vi "DataQuery.vi"(8 "Error In":errorcluster, 11 "Configur.Database Configuration":T1) -> (0 "Error Out":errorcluster)   [LabVIEW 2025, in "Full User Interface.lvlib"]
uses:
  Full User Interface.lvlib
  <vilib>/Test Bench Framework/Test Executive.lvlibp/TestEngine/TestEngine/TestEngine/Typedefs/Database Configuration.ctl
  <vilib>/Test Bench Framework/Query Data(Serial Number).vi
  <vilib>/Test Bench Framework/Query Data(Time Range).vi
  <vilib>/Test Bench Framework/Test Executive(API).lvlib
  <vilib>/Utility/sysdir.llb/System Directory Type.ctl
  <vilib>/Test Bench Framework/Query Data(Export).vi
  <vilib>/Test Bench Framework/Test Executive.lvlibp/TestEngine/TestEngine/TestEngine/Test Engine.lvclass
panel:
  in  "Query":bool
  in  "Serial Number":string caption="产品序列号"
  in  "End Time":timestamp caption="结束时间" format="%<%x %.3X>T"
  in  "Start Time":timestamp caption="起始时间" format="%<%x %.3X>T"
  in  "Sequence Name":string caption="表格（序列文件名）"
  in  "Listbox":i32(listbox)
  in  "Export":bool
  in  "Page":i32 min=0 max=1000 format="Page: %d"
  in  "Next":bool
  in  "Previous":bool
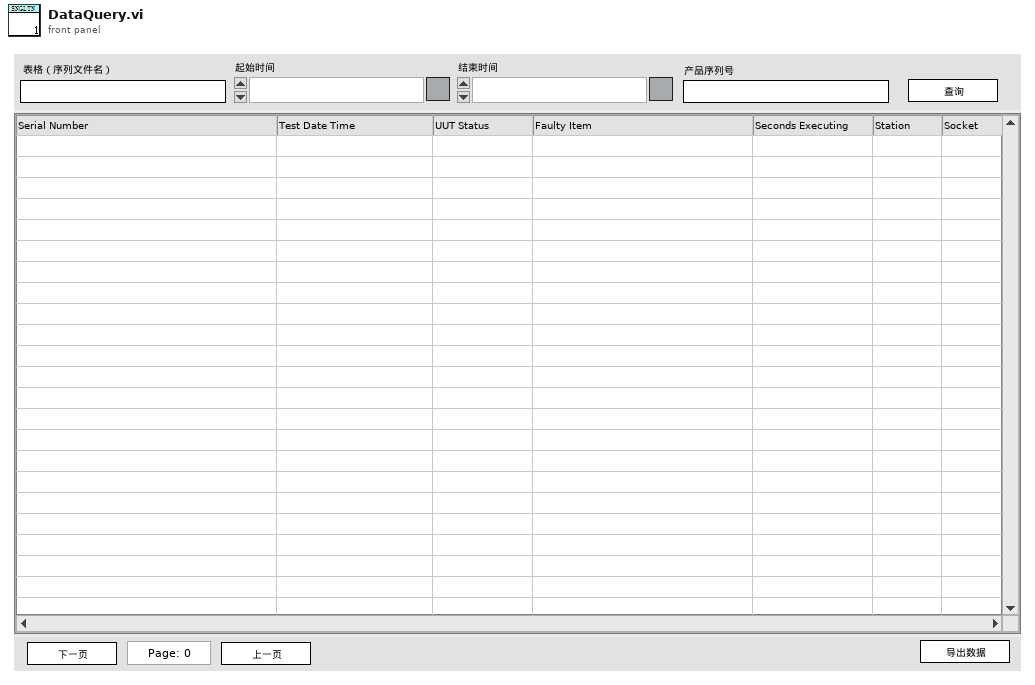
[diagram p1: front panel]
types:
  T1 = typedef "Test Executive.lvlibp/Test Engine.lvlib/Test Engine.lvclass/Database Configuration.ctl" = cluster{"Connection String Expression":string, "Microsoft Data Link File":path, "Connection Type":enum16{"Use Connection String Expression", "Use Microsoft Data Link File"}, "Enable":bool}
  T2 = enum32{"Invalid", "Standard", "Closed", "Hidden", "Minimized", "Maximized"}
  T3 = enum32{"invalid app kind", "Development System", "Run Time System", "Student Edition", "Embedded LabVIEW", "Evaluation", "Custom"}
  T4 = cluster{"Core":cluster{"Current VI Reference":refnum<vi>, "Close Panel on Exit?":bool}, "Listbox":refnum<vi>, "Serial Number":refnum<vi>, "Start Time":refnum<vi>, "End Time":refnum<vi>, "Sequence Name":refnum<vi>, "Data":cluster{"Cluster":cluster{"General":cluster{"Sequence Name":string, "Serial Number":string, "Test Date Time":string, "UUT Status":string, "Faulty Item":string, "Seconds Executing":string}, "Tree Control Items":cluster{"Left Cell String":string, "Child Text":string[], "Child Tag":string, "Item Indent":i32, "Child Only?":bool, "Glyph Index":i32}[]}, "Station":string, "Socket":i32}[], "Page":refnum<vi>}
  T5 = cluster{"Cluster":cluster{"General":cluster{"Sequence Name":string, "Serial Number":string, "Test Date Time":string, "UUT Status":string, "Faulty Item":string, "Seconds Executing":string}, "Tree Control Items":cluster{"Left Cell String":string, "Child Text":string[], "Child Tag":string, "Item Indent":i32, "Child Only?":bool, "Glyph Index":i32}[]}, "Station":string, "Socket":i32}[]
  T6 = cluster{"Current VI Reference":refnum<vi>, "Close Panel on Exit?":bool}
  T7 = cluster{"Cluster":cluster{"General":cluster{"Sequence Name":string, "Serial Number":string, "Test Date Time":string, "UUT Status":string, "Faulty Item":string, "Seconds Executing":string}, "Tree Control Items":cluster{"Left Cell String":string, "Child Text":string[], "Child Tag":string, "Item Indent":i32, "Child Only?":bool, "Glyph Index":i32}[]}, "Station":string, "Socket":i32}
  T8 = typedef "System Directory Type.ctl" = i32
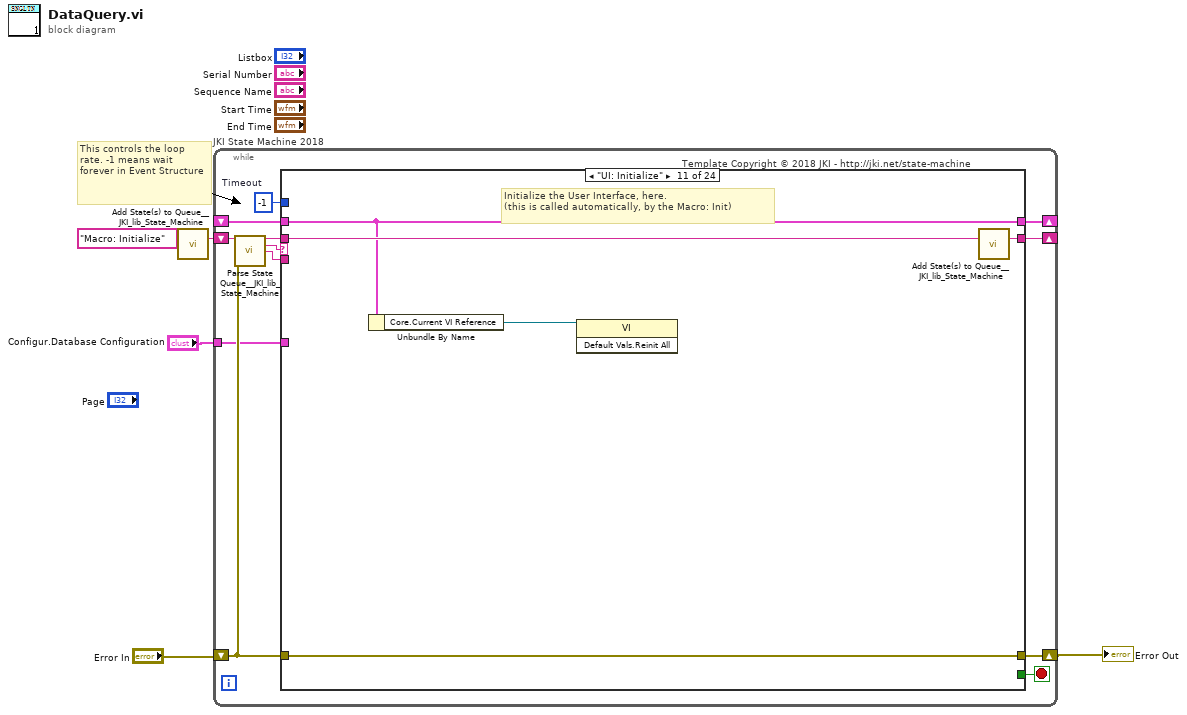
[diagram p0: block diagram]
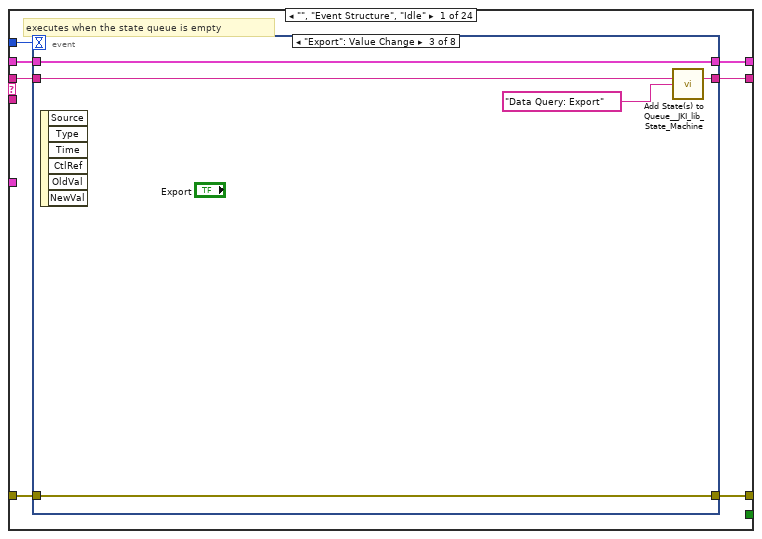
[diagram p2: hidden frame]
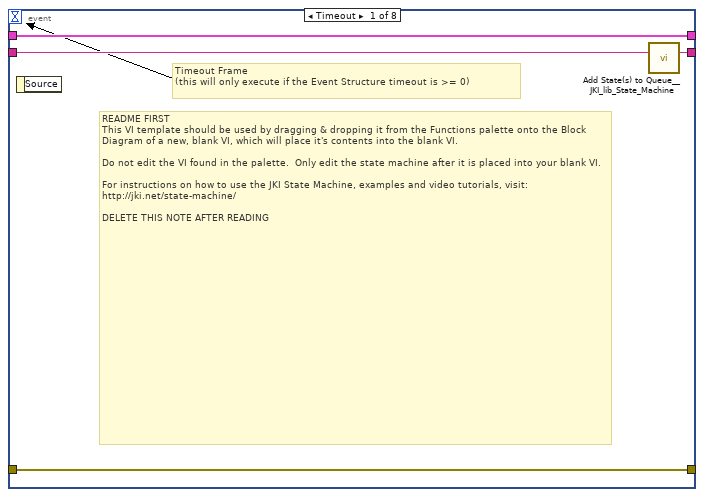
[diagram p3: hidden frame]
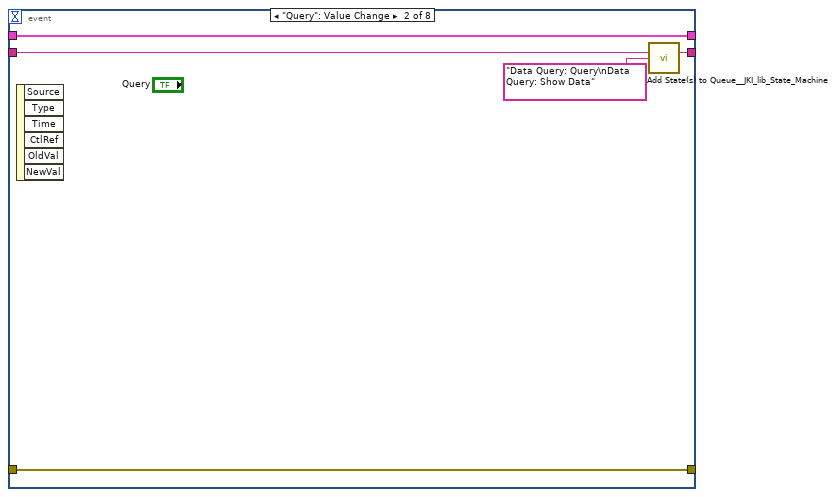
[diagram p4: hidden frame]
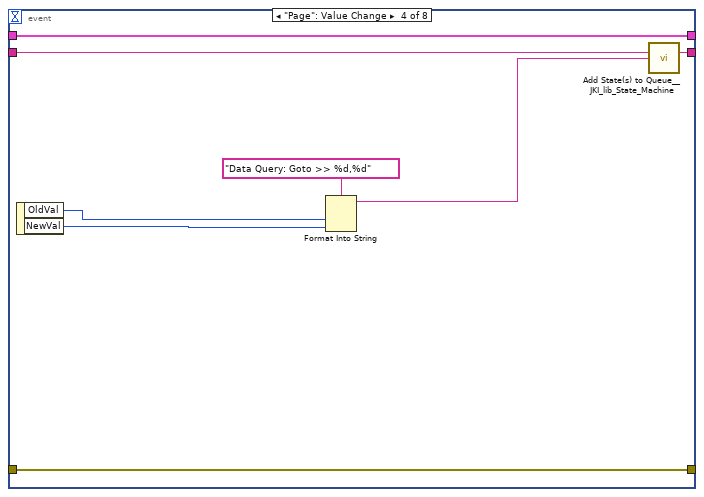
[diagram p5: hidden frame]
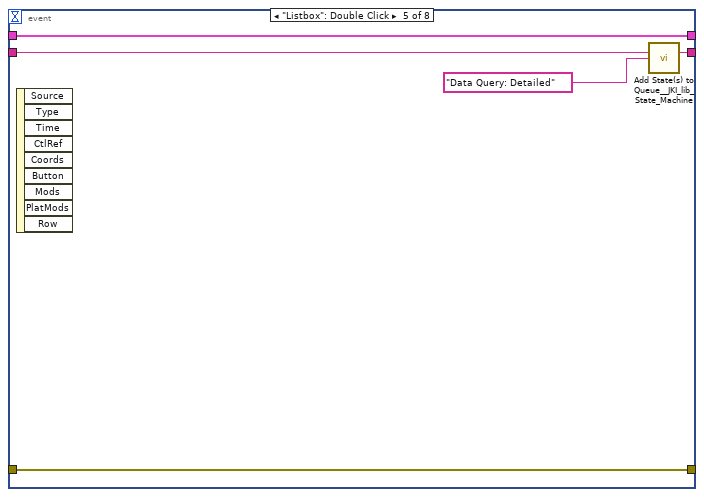
[diagram p6: hidden frame]
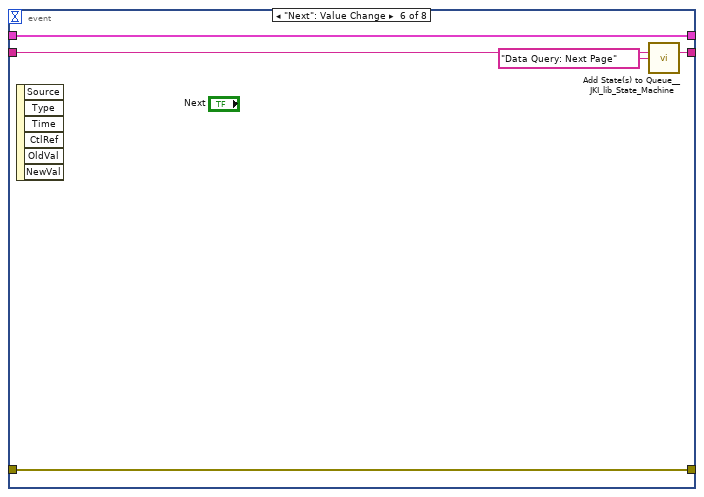
[diagram p7: hidden frame]
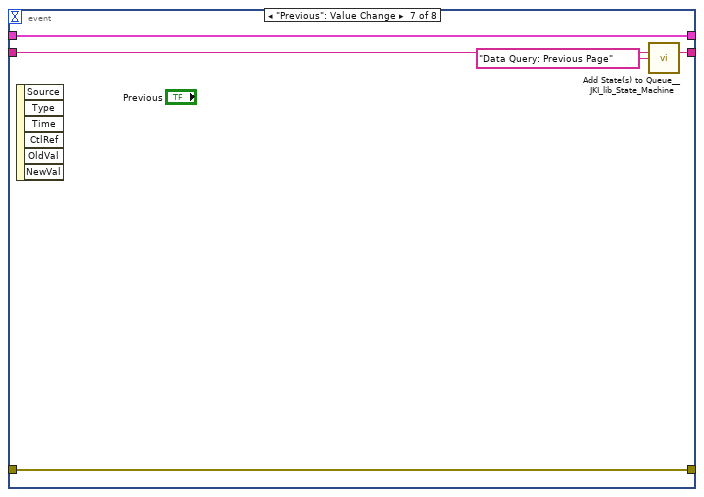
[diagram p8: hidden frame]
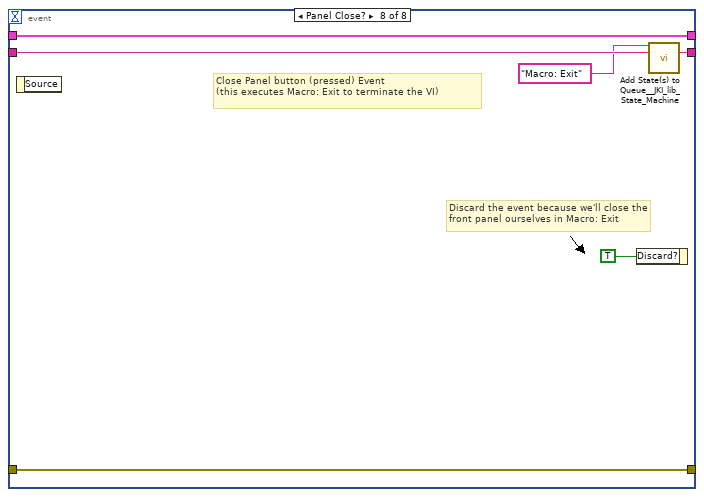
[diagram p9: hidden frame]
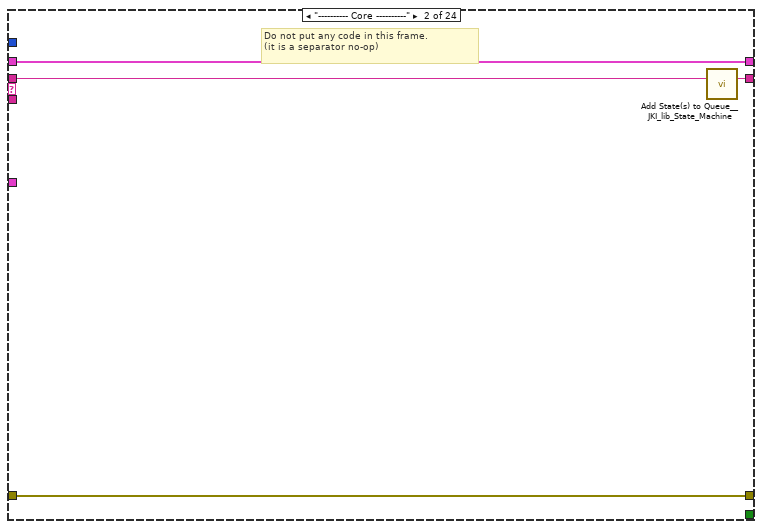
[diagram p10: hidden frame]
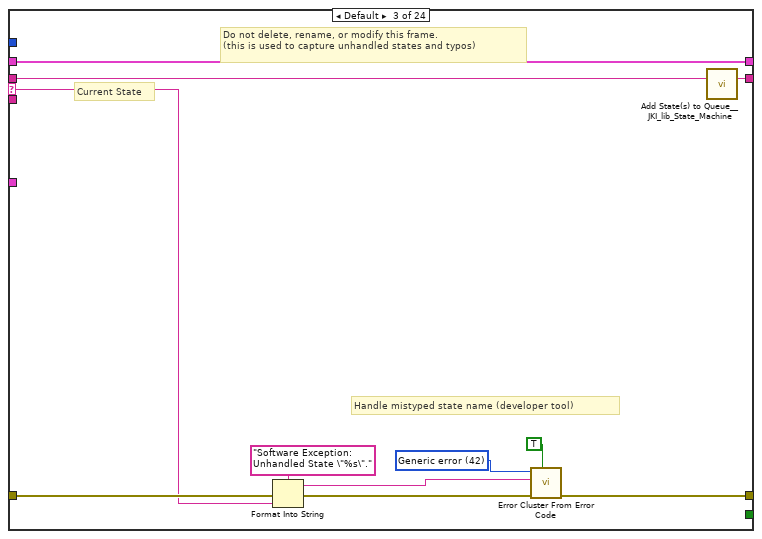
[diagram p11: hidden frame]
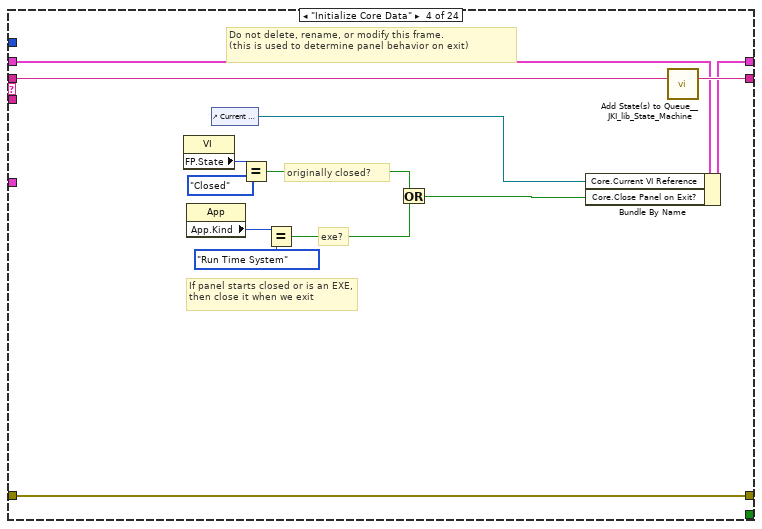
[diagram p12: hidden frame]
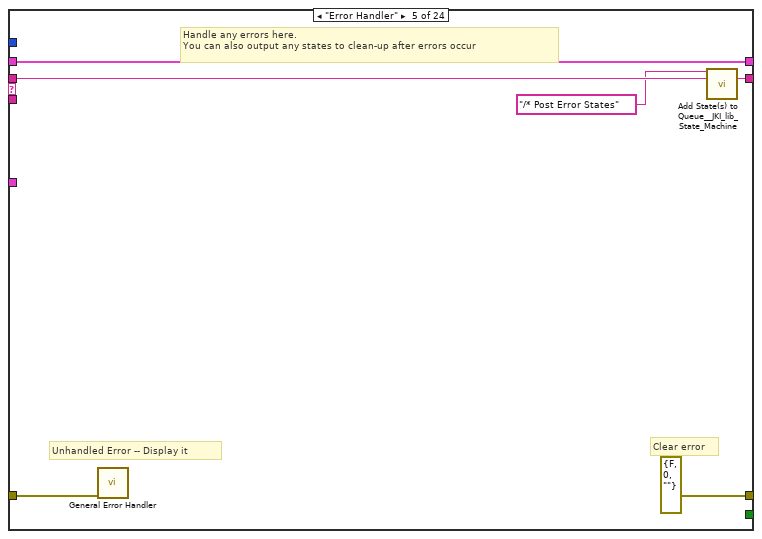
[diagram p13: hidden frame]
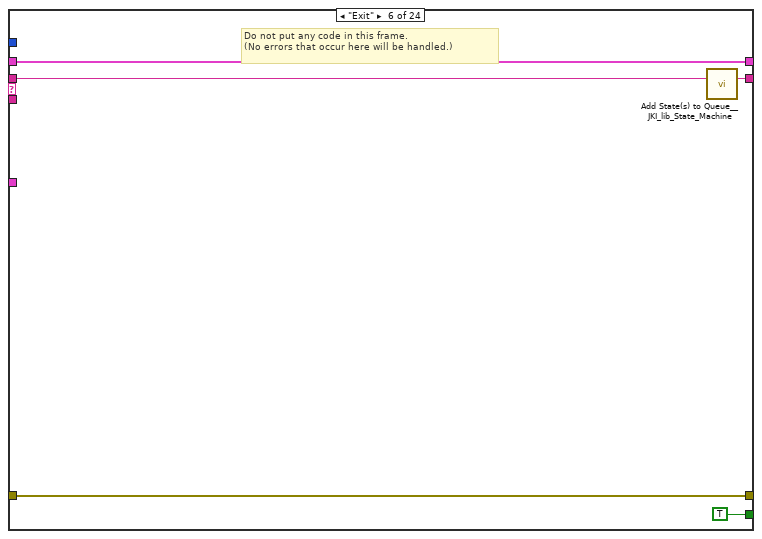
[diagram p14: hidden frame]
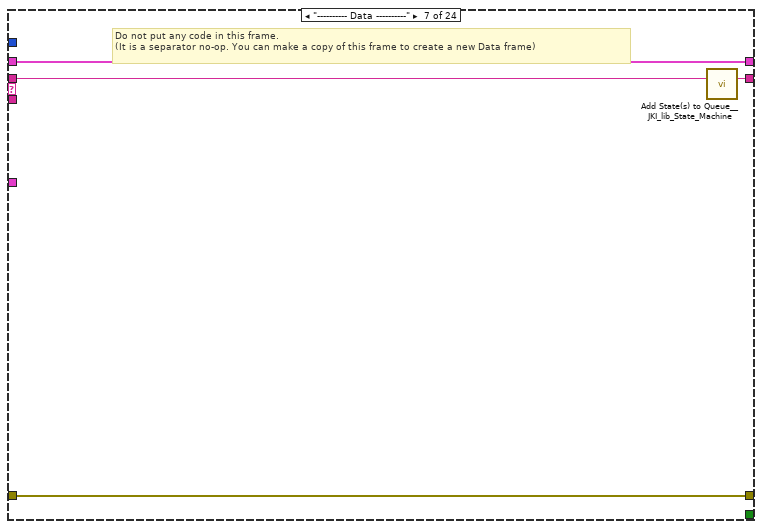
[diagram p15: hidden frame]
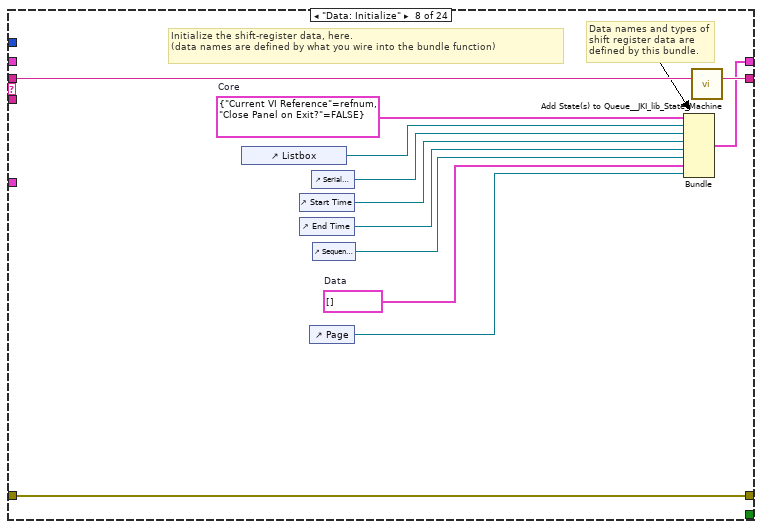
[diagram p16: hidden frame]
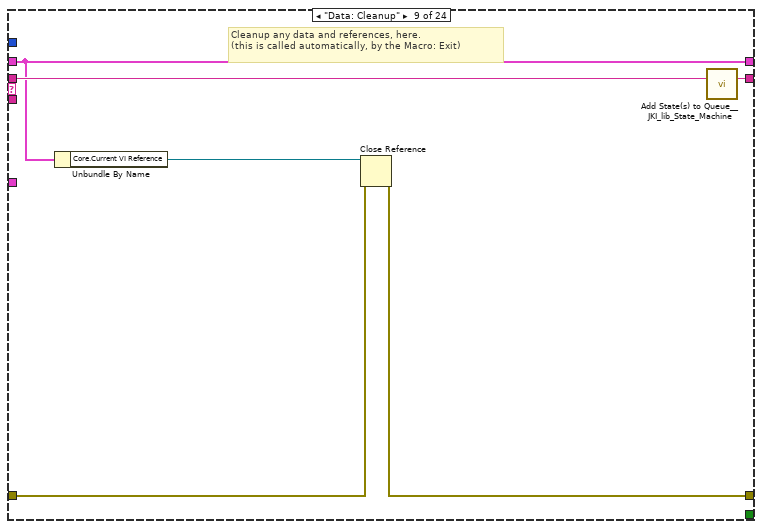
[diagram p17: hidden frame]
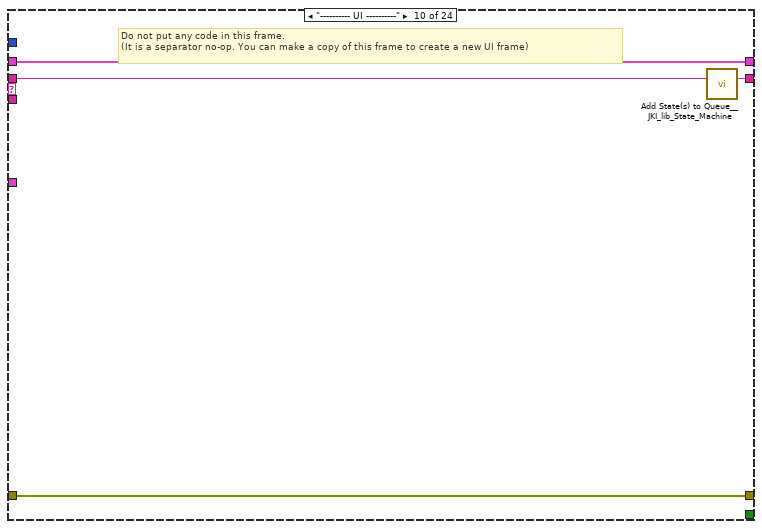
[diagram p18: hidden frame]
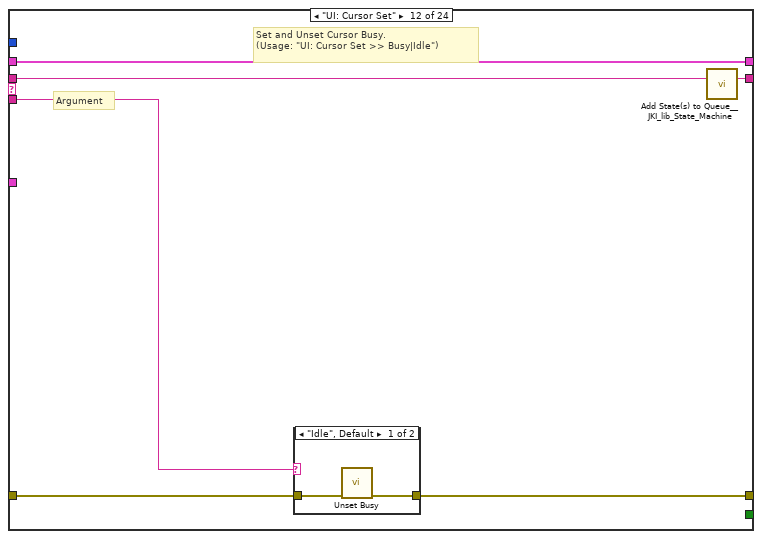
[diagram p19: hidden frame]
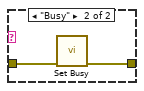
[diagram p20: hidden frame]
diagram:
  # "This controls the loop rate. -1 means wait forever in Event Structure"
  n1 = call <vilib>:"Add State(s) to Queue__JKI_lib_State_Machine.vi"("State(s) in (\"\")"="Macro: Initialize") -> ("States Out"=w5:string)  [unwired: 14 in]
  n2 = while "JKI State Machine 2018" {
    shift-right: [w10] -> _
    shift-left: _ -> [w9]
    shift-right: [w13] -> w3
    shift-left: "Error In" -> [w7]
    shift-right: [w12] -> _
    shift-left: w5 -> [w14]
    tunnel: "Configur.Database Configuration" -> [w6]
    stop <- w11 stop-if-true
    w8 = -1  # Timeout
    # "Template Copyright © 2018 JKI - http://jki.net/state-machine"
    n3 = call <vilib>:"Parse State Queue__JKI_lib_State_Machine.vi"("State Queue"=w14, "Error In (no error)"=w7) -> ("Remaining States"=w16:string, "Current State"=w17:string, "Arguments"=w15:string)  [unwired: 11 in]
    n4 = case shown="\"UI: Initialize\"" w17 {
      selector: w17 -> [_ _ w72 _ _ _ _ _ _ _ _ _ _ _ _ _ _ _ _ _ _ _ _ _]
      tunnel: w16 -> [w24 w71 w76 w95 w101 w106 w110 w122 w128 w132 w137 w143 w154 w223 w228 w238 w242 w261 w280 w302 w320 w333 w340 w371]
      tunnel: w15 -> [_ _ _ _ _ _ _ _ _ _ _ w138 w148 _ _ _ _ _ _ _ _ _ _ w359]
      tunnel: w9 -> [w22 w68 w74 w88 w98 w104 w107 _ w123 w129 w134 w141 w150 w220 w225 w235 w239 w247 w277 w299 w317 w327 w337 w363]
      tunnel: [w21 w69 w78 w92 errorcluster {"status"=FALSE, "code"=0, "source"=""} ("error out") w103 w108 w119 w124 w130 w135 w139 w151 w221 w226 w236 w240 w259 w278 w300 w318 w331 w338 w369] -> w13
      tunnel: w7 -> [w20 w69 w77 w92 w97 w103 w108 w119 w125 w130 w135 w140 w152 w221 w226 w236 w240 w259 w278 w300 w318 w331 w338 w369]
      tunnel: [w23 w70 w75 w94 w100 w105 w109 w121 w127 w131 w136 w142 w153 w222 w227 w237 w241 w260 w279 w301 w319 w332 w339 w370] -> w12
      tunnel: [_ _ _ _ _ TRUE _ _ _ _ _ _ _ _ _ _ _ _ _ _ _ _ _ _] -> w11
      tunnel: [w19 w68 w74 w93 w98 w104 w107 w120 w123 w129 w134 w141 w150 w220 w225 w235 w239 w245 w277 w299 w317 w327 w337 w363] -> w10
      tunnel: w8 -> [w18 _ _ _ _ _ _ _ _ _ _ _ _ _ _ _ _ _ _ _ _ _ _ _]
      tunnel: w6 -> [_ _ _ _ _ _ _ _ _ _ _ _ _ _ _ _ _ w258 _ _ _ _ _ _]
      frame "", "Event Structure", "Idle" {
        # "executes when the state queue is empty"
        n5 = event shown="[2] \"Export\": Value Change" {
          selector: _ -> [_ _ _ _ _ _ _ _]
          dyn-events: _ -> [_ _ _ _ _ _ _ _]
          timeout: w18 -> [_ _ _ _ _ _ _ _]
          tunnel: w24 -> [w28 w33 w38 w46 w51 w56 w61 w67]
          tunnel: [w27 w32 w37 w45 w50 w55 w60 w66] -> w23
          tunnel: w22 -> [w25 w30 w35 w43 w48 w53 w58 w64]
          tunnel: [w26 w31 w36 w44 w49 w54 w59 w65] -> w21
          tunnel: w20 -> [w26 w31 w36 w44 w49 w54 w59 w65]
          tunnel: [w25 w30 w35 w43 w48 w53 w58 w64] -> w19
          event Timeout {
            # "README FIRST\nThis VI template should be used by dragging & dropping it from the Functions palette onto the Block Diagram of a new, blank VI, which will place it's contents into the blank VI.\n\nDo not edit the VI found in the palette.  Only edit the state machine after it is placed into your blank VI.\n\nFor instructions on how to use the JKI State Machine, examples and video tutorials, visit:\nhttp://jki.net/state-machine/\n\nDELETE THIS NOTE AFTER READING"
            # "Timeout Frame\n(this will only execute if the Event Structure timeout is >= 0)"
            n6 = event-data() -> ()  [unwired: 1 in, 1 out]
            n7 = call <vilib>:"Add State(s) to Queue__JKI_lib_State_Machine.vi"("State(s) in (\"\")"=w28) -> ("States Out"=w27:string)  [unwired: 14 in]
          }
          event "Query": Value Change {
            n8 = event-data() -> ()  [unwired: 1 in, 6 out]
            n9 = call <vilib>:"Add State(s) to Queue__JKI_lib_State_Machine.vi"("State(s) in (\"\")"=w33, "State(s) at Back (\"\")"="Data Query: Query\nData Query: Show Data" ("State(s) at Back (\"\")")) -> ("States Out"=w32:string)  [unwired: 13 in]
          }
          event "Export": Value Change {
            n10 = event-data() -> ()  [unwired: 1 in, 6 out]
            n11 = call <vilib>:"Add State(s) to Queue__JKI_lib_State_Machine.vi"("State(s) in (\"\")"=w38, "State(s) at Back (\"\")"="Data Query: Export" ("State(s) at Back (\"\")")) -> ("States Out"=w37:string)  [unwired: 13 in]
          }
          event "Page": Value Change {
            n12 = event-data() -> ("OldVal"=w40:i32, "NewVal"=w39:i32)  [unwired: 1 in]
            n13 = Format Into String(format string="Data Query: Goto >> %d,%d", w40, w39) -> (resulting string=w41:string)  [unwired: 2 in, 1 out]
            n14 = call <vilib>:"Add State(s) to Queue__JKI_lib_State_Machine.vi"("State(s) in (\"\")"=w46, "State(s) at Back (\"\")"=w41) -> ("States Out"=w45:string)  [unwired: 13 in]
          }
          event "Listbox": Double Click {
            n15 = event-data() -> ()  [unwired: 1 in, 9 out]
            n16 = call <vilib>:"Add State(s) to Queue__JKI_lib_State_Machine.vi"("State(s) in (\"\")"=w51, "State(s) at Back (\"\")"="Data Query: Detailed" ("State(s) at Back (\"\")")) -> ("States Out"=w50:string)  [unwired: 13 in]
          }
          event "Next": Value Change {
            n17 = event-data() -> ()  [unwired: 1 in, 6 out]
            n18 = call <vilib>:"Add State(s) to Queue__JKI_lib_State_Machine.vi"("State(s) in (\"\")"=w56, "State(s) at Back (\"\")"="Data Query: Next Page" ("State(s) at Back (\"\")")) -> ("States Out"=w55:string)  [unwired: 13 in]
          }
          event "Previous": Value Change {
            n19 = event-data() -> ()  [unwired: 1 in, 6 out]
            n20 = call <vilib>:"Add State(s) to Queue__JKI_lib_State_Machine.vi"("State(s) in (\"\")"=w61, "State(s) at Back (\"\")"="Data Query: Previous Page" ("State(s) at Back (\"\")")) -> ("States Out"=w60:string)  [unwired: 13 in]
          }
          event Panel Close? {
            # "Discard the event because we'll close the front panel ourselves in Macro: Exit"
            # "Close Panel button (pressed) Event\n(this executes Macro: Exit to terminate the VI)"
            n21 = event-data() -> ()  [unwired: 1 in, 1 out]
            n22 = event-data("Discard?"=TRUE) -> ()  [unwired: 1 in, 1 out]
            n23 = call <vilib>:"Add State(s) to Queue__JKI_lib_State_Machine.vi"("State(s) in Front (\"\")"="Macro: Exit", "State(s) in (\"\")"=w67) -> ("States Out"=w66:string)  [unwired: 13 in]
          }
        }
      }
      frame "---------- Core ----------" {
        # "Do not put any code in this frame.\n(it is a separator no-op)"
        n24 = call <vilib>:"Add State(s) to Queue__JKI_lib_State_Machine.vi"("State(s) in (\"\")"=w71) -> ("States Out"=w70:string)  [unwired: 14 in]
      }
      frame Default {
        w81 = 42 items=["No error", "Argument error", "Memory is full", "Out of zone", "End of file", "File already open", "Generic file I/O error", "File not found", "File permission error", "Disk is full", "Duplicate path", "Too many files open", "System feature not enabled", "Resource file not found", "Cannot add resource", "Resource not found", "Image not found", "Image memory error", "Pen does not exist", "Config type invalid", "Config token not found", "Config parse error", "Config memory error", "Bad external code format", "Bad external code offset", "External code not present", "Null window", "Destroy window error", "Null menu", "Print aborted", "Bad print record", "Print driver error", "Windows error during printing", "Memory error during printing", "Print dialog error", "Generic print error", "Invalid device refnum", "Device not found", "Device parameter error", "Device unit error", "Cannot open device", "Device call aborted", "Generic error", "Cancelled by user", "Object ID too low", "Object ID too high", "Object not in heap", "Unknown heap", "Unknown object (invalid DefProc)", "Unknown object (DefProc not in table)", "Message out of range", "Invalid (null) method", "Unknown message", "Manager call not supported", "Bad address", "Network operation in progress", "Network operation timed out", "Connection is busy", "Network attribute not supported", "Network error", "Address in use", "System out of memory", "Connection aborted", "Connection refused", "Not connected", "Already connected", "Connection closed", "Initialization error (interapplication manager)", "Bad occurrence", "Wait on unbound occurrence handler", "Occurrence queue overflow", "Datalog type conflict", "Unused", "Unrecognized type (interapplication manager)", "Memory corrupt", "Failed to make temporary DLL", "Old CIN version", "Drag socket not found", "Failed to load drop-object", "Failed to register OLE object", "Failed to release OLE object", "Format specifier type mismatch", "Unknown format specifier", "Too few format specifiers", "Too many format specifiers", "Scan failed", "Newer CIN version", "Error converting to variant", "Runtime menu error", "Password tampered", "Variant attribute not found", "Incompatible variant data type", "Event data is not available", "Event Store is not present", "Occurrence is not found", "Event Queue is not created", "Event info is not available", "Refnum passed is NULL", "Error retrieving Class GUID", "Error retrieving CoClass GUID", "Error retrieving TypeLib GUID.", "Bad built application magic bytes.", "Specific driver is different from the specific driver associated with the Logical Name.", "There is no session opened to the class driver.", "Max Error", "MAX - Error with config objects", "MAX - Error loading configuration", "MAX - Group not supported"]
        # "Current State"
        # "Do not delete, rename, or modify this frame.\n(this is used to capture unhandled states and typos)"
        # "Handle mistyped state name (developer tool)"
        n25 = Format Into String(format string="Software Exception: Unhandled State \"%s\"." ("message"), error in=w77, w72) -> (resulting string=w80:string, error out=w79:errorcluster)  [unwired: 1 in]
        n26 = call <vilib>:"Error Cluster From Error Code.vi"("show call chain? (False)"=TRUE, "error in (no error)"=w79, "error message (\"\")"=w80, "error code (0)"=w81) -> ("error out"=w78:errorcluster)  [unwired: 5 in]
        n27 = call <vilib>:"Add State(s) to Queue__JKI_lib_State_Machine.vi"("State(s) in (\"\")"=w76) -> ("States Out"=w75:string)  [unwired: 14 in]
      }
      frame "Initialize Core Data" {
        # "Do not delete, rename, or modify this frame.\n(this is used to determine panel behavior on exit)"
        # "originally closed?"
        # "exe?"
        # "If panel starts closed or is an EXE, then close it when we exit"
        n28 = property class="VI"() -> ("FP.State"=w85:T2)  [unwired: 2 in, 2 out]
        n29 = property class="App"() -> ("App.Kind"=w91:T3)  [unwired: 2 in, 2 out]
        n30 = control-ref of="Current VI Reference"() -> (w86:refnum<vi>)
        n31 = Equal?(x=w85, y=T2."Closed" ("Front Panel Window:State")) -> (x = y?=w83:bool)
        n32 = Equal?(x=w91, y=T3."Run Time System" ("Application:Kind")) -> (x = y?=w89:bool)
        n33 = Or(x=w83, y=w89) -> (x .or. y?=w87:bool)
        n34 = Bundle By Name(cluster=w88, "Core.Current VI Reference"=w86, "Core.Close Panel on Exit?"=w87) -> (w93:T4)
        n35 = call <vilib>:"Add State(s) to Queue__JKI_lib_State_Machine.vi"("State(s) in (\"\")"=w95) -> ("States Out"=w94:string)  [unwired: 14 in]
      }
      frame "Error Handler" {
        # "Unhandled Error -- Display it"
        # "Handle any errors here.\nYou can also output any states to clean-up after errors occur"
        # "Clear error"
        n36 = call <vilib>:"General Error Handler.vi"("error in (no error)"=w97) -> ()  [unwired: 10 in, 5 out]
        n37 = call <vilib>:"Add State(s) to Queue__JKI_lib_State_Machine.vi"("State(s) in Front (\"\")"="/* Post Error States", "State(s) in (\"\")"=w101) -> ("States Out"=w100:string)  [unwired: 13 in]
      }
      frame "Exit" {
        # "Do not put any code in this frame.\n(No errors that occur here will be handled.)"
        n38 = call <vilib>:"Add State(s) to Queue__JKI_lib_State_Machine.vi"("State(s) in (\"\")"=w106) -> ("States Out"=w105:string)  [unwired: 14 in]
      }
      frame "---------- Data ----------" {
        # "Do not put any code in this frame.\n(It is a separator no-op. You can make a copy of this frame to create a new Data frame)"
        n39 = call <vilib>:"Add State(s) to Queue__JKI_lib_State_Machine.vi"("State(s) in (\"\")"=w110) -> ("States Out"=w109:string)  [unwired: 14 in]
      }
      frame "Data: Initialize" {
        w112 = T5 []  # Data
        w118 = T6 {"Current VI Reference"=refnum, "Close Panel on Exit?"=FALSE}  # Core
        # "Data names and types of shift register data are defined by this bundle."
        # "Initialize the shift-register data, here.\n(data names are defined by what you wire into the bundle function)"
        n40 = control-ref of="Listbox"() -> (w117:refnum<vi>)
        n41 = control-ref of="Start Time"() -> (w115:refnum<vi>)
        n42 = control-ref of="End Time"() -> (w114:refnum<vi>)
        n43 = control-ref of="Page"() -> (w111:refnum<vi>)
        n44 = control-ref of="Serial Number"() -> (w116:refnum<vi>)
        n45 = control-ref of="Sequence Name"() -> (w113:refnum<vi>)
        n46 = Bundle("Core"=w118, "Listbox"=w117, "Serial Number"=w116, "Start Time"=w115, "End Time"=w114, "Sequence Name"=w113, "Data"=w112, "Page"=w111) -> (w120:T4)  [unwired: 1 in]
        n47 = call <vilib>:"Add State(s) to Queue__JKI_lib_State_Machine.vi"("State(s) in (\"\")"=w122) -> ("States Out"=w121:string)  [unwired: 14 in]
      }
      frame "Data: Cleanup" {
        # "Cleanup any data and references, here.\n(this is called automatically, by the Macro: Exit)"
        n48 = Unbundle By Name(w123) -> ("Core.Current VI Reference"=w126:refnum<vi>)
        n49 = Close Reference(reference=w126, error in (no error)=w125) -> (error out=w124:errorcluster)
        n50 = call <vilib>:"Add State(s) to Queue__JKI_lib_State_Machine.vi"("State(s) in (\"\")"=w128) -> ("States Out"=w127:string)  [unwired: 14 in]
      }
      frame "---------- UI ----------" {
        # "Do not put any code in this frame.\n(It is a separator no-op. You can make a copy of this frame to create a new UI frame)"
        n51 = call <vilib>:"Add State(s) to Queue__JKI_lib_State_Machine.vi"("State(s) in (\"\")"=w132) -> ("States Out"=w131:string)  [unwired: 14 in]
      }
      frame "UI: Initialize" {
        # "Initialize the User Interface, here.\n(this is called automatically, by the Macro: Init)"
        n52 = Unbundle By Name(w134) -> ("Core.Current VI Reference"=w133:refnum<vi>)
        n53 = invoke class="VI" method="Default Vals.Reinit All"(reference=w133) -> ()  [unwired: 2 in, 3 out]
        n54 = call <vilib>:"Add State(s) to Queue__JKI_lib_State_Machine.vi"("State(s) in (\"\")"=w137) -> ("States Out"=w136:string)  [unwired: 14 in]
      }
      frame "UI: Cursor Set" {
        # "Argument"
        # "Set and Unset Cursor Busy.\n(Usage: \"UI: Cursor Set >> Busy|Idle\")"
        n55 = case shown="\"Idle\", Default" w138 {
          tunnel: w140 -> [w145 w147]
          tunnel: [w144 w146] -> w139
          frame "Idle", Default {
            n56 = call <vilib>:"Unset Busy.vi"("error in (no error)"=w145) -> ("error out"=w144:errorcluster)  [unwired: 10 in]
          }
          frame "Busy" {
            n57 = call <vilib>:"Set Busy.vi"("error in (no error)"=w147) -> ("error out"=w146:errorcluster)  [unwired: 9 in, 1 out]
          }
        }
        n58 = call <vilib>:"Add State(s) to Queue__JKI_lib_State_Machine.vi"("State(s) in (\"\")"=w143) -> ("States Out"=w142:string)  [unwired: 14 in]
      }
      frame "UI: Front Panel State" {
        # "Argument"
        # "Set Front Panel Open or Closed\n(Usage: \"UI: Front Panel State >> Open|Close\")"
        n59 = Unbundle By Name(w150) -> ("Core.Current VI Reference"=w149:refnum<vi>)
        n60 = case shown="\"Minimize\", \"Minimized\"" w148 {
          tunnel: w152 -> [w160 w175 w186 w199 w212]
          tunnel: [w162 w176 w188 w201 w214] -> w151
          tunnel: w149 -> [w161 w173 w187 w200 w213]
          frame "Open", "Standard", Default {
            w155 = T2."Standard" ("State")
            n61 = property class="VI"(reference=w161, error in=w160) -> (reference out=w158:refnum<vi>, error out=w159:errorcluster, "FP.State"=w157:T2)
            n62 = Not Equal?(x=w157, y=w155) -> (x != y?=w156:bool)
            n63 = case shown="True" w156 {
              tunnel: [w166 w168] -> w162
              tunnel: w159 -> [w165 w168]
              tunnel: w158 -> [w164 _]
              tunnel: w155 -> [w163 _]
              frame True {
                n64 = invoke class="VI" method="FP.Open"(reference=w164, error in=w165, "Activate"=TRUE, "State"=w163) -> (error out=w166:errorcluster)  [unwired: 1 in, 4 out]
              }
              frame False {
              }
            }
          }
          frame "Close", "Closed" {
            n65 = property class="VI"(reference=w173, error in=w175) -> (reference out=w172:refnum<vi>, error out=w174:errorcluster, "FP.State"=w170:T2)
            n66 = Not Equal?(x=w170, y=T2."Closed" ("Front Panel Window:State")) -> (x != y?=w169:bool)
            n67 = case shown="True" w169 {
              tunnel: [w177 w180] -> w176
              tunnel: w174 -> [w177 w179]
              tunnel: w172 -> [_ w178]
              frame False {
              }
              frame True {
                n68 = invoke class="VI" method="FP.Close"(reference=w178, error in=w179) -> (error out=w180:errorcluster)  [unwired: 1 in, 2 out]
              }
            }
          }
          frame "Hidden", "Hide" {
            w181 = T2."Hidden" ("State")
            n69 = property class="VI"(reference=w187, error in=w186) -> (reference out=w184:refnum<vi>, error out=w185:errorcluster, "FP.State"=w183:T2)
            n70 = Not Equal?(x=w183, y=w181) -> (x != y?=w182:bool)
            n71 = case shown="True" w182 {
              tunnel: [w192 w193] -> w188
              tunnel: w185 -> [w191 w193]
              tunnel: w184 -> [w190 _]
              tunnel: w181 -> [w189 _]
              frame True {
                n72 = invoke class="VI" method="FP.Open"(reference=w190, error in=w191, "State"=w189) -> (error out=w192:errorcluster)  [unwired: 2 in, 4 out]
              }
              frame False {
              }
            }
          }
          frame "Minimize", "Minimized" {
            w194 = T2."Minimized" ("State")
            n73 = property class="VI"(reference=w200, error in=w199) -> (reference out=w197:refnum<vi>, error out=w198:errorcluster, "FP.State"=w196:T2)
            n74 = Not Equal?(x=w196, y=w194) -> (x != y?=w195:bool)
            n75 = case shown="True" w195 {
              tunnel: [w205 w206] -> w201
              tunnel: w198 -> [w204 w206]
              tunnel: w197 -> [w203 _]
              tunnel: w194 -> [w202 _]
              frame True {
                n76 = invoke class="VI" method="FP.Open"(reference=w203, error in=w204, "State"=w202) -> (error out=w205:errorcluster)  [unwired: 2 in, 4 out]
              }
              frame False {
              }
            }
          }
          frame "Maximize", "Maximized" {
            w207 = T2."Maximized" ("State")
            n77 = property class="VI"(reference=w213, error in=w212) -> (reference out=w210:refnum<vi>, error out=w211:errorcluster, "FP.State"=w209:T2)
            n78 = Not Equal?(x=w209, y=w207) -> (x != y?=w208:bool)
            n79 = case shown="True" w208 {
              tunnel: [w218 w219] -> w214
              tunnel: w211 -> [w217 w219]
              tunnel: w210 -> [w216 _]
              tunnel: w207 -> [w215 _]
              frame True {
                n80 = invoke class="VI" method="FP.Open"(reference=w216, error in=w217, "State"=w215) -> (error out=w218:errorcluster)  [unwired: 2 in, 4 out]
              }
              frame False {
              }
            }
          }
        }
        n81 = call <vilib>:"Add State(s) to Queue__JKI_lib_State_Machine.vi"("State(s) in (\"\")"=w154) -> ("States Out"=w153:string)  [unwired: 14 in]
      }
      frame "---------- Macro ----------" {
        # "Do not put any code in this frame.\n(It is a separator no-op. You can make a copy of this frame to create a new Macro frame)"
        n82 = call <vilib>:"Add State(s) to Queue__JKI_lib_State_Machine.vi"("State(s) in (\"\")"=w223) -> ("States Out"=w222:string)  [unwired: 14 in]
      }
      frame "Macro: Initialize" {
        w224 = "Data: Initialize\nInitialize Core Data\nUI: Initialize\nUI: Front Panel State >> Open"  # Data: Initialize Initialize Core Data UI: Initialize UI: Front Panel State >> Open
        # "Initialization Macro\n(This is called once, when the VI starts)"
        n83 = call <vilib>:"Add State(s) to Queue__JKI_lib_State_Machine.vi"("State(s) in Front (\"\")"=w224, "State(s) in (\"\")"=w228) -> ("States Out"=w227:string)  [unwired: 13 in]
      }
      frame "Macro: Exit" {
        # "Exit Macro\n(This is called once, when the VI exits)"
        n84 = Unbundle By Name(w235) -> ("Core.Close Panel on Exit?"=w234:bool)
        n85 = Select(t="UI: Front Panel State >> Close", s=w234, f="") -> (s? t:f=w231:string)
        n86 = call <vilib>:"Add State(s) to Queue__JKI_lib_State_Machine.vi"("State(s) in (\"\")"=w231, "State(s) at Back (\"\")"="Data: Cleanup\nExit") -> ("States Out"=w229:string)  [unwired: 13 in]
        n87 = call <vilib>:"Add State(s) to Queue__JKI_lib_State_Machine.vi"("State(s) in Front (\"\")"=w229, "State(s) in (\"\")"=w238) -> ("States Out"=w237:string)  [unwired: 13 in]
      }
      frame "---------- Data Query ----------" {
        # "Template Separator\n(You can make a copy of, or modify, this frame)"
        n88 = call <vilib>:"Add State(s) to Queue__JKI_lib_State_Machine.vi"("State(s) in (\"\")"=w242) -> ("States Out"=w241:string)  [unwired: 14 in]
      }
      frame "Data Query: Query" {
        # "Your code here.\n(You can make a copy of, or modify, this frame)"
        n89 = Unbundle By Name(w247) -> ("Start Time"=w255:refnum<vi>, "End Time"=w254:refnum<vi>, "Sequence Name"=w257:refnum<vi>, "Serial Number"=w250:refnum<vi>, "Page"=w244:refnum<vi>)
        n90 = property class="AbsTime (strict)"(reference=w255) -> ("Value"=w253:timestamp)  [unwired: 1 in, 2 out]
        n91 = property class="AbsTime (strict)"(reference=w254) -> ("Value"=w252:timestamp)  [unwired: 1 in, 2 out]
        n92 = property class="Str"(reference=w257) -> ("Value"=w256:string)  [unwired: 1 in, 2 out]
        n93 = property class="Str"(reference=w250) -> ("Value"=w248:string)  [unwired: 1 in, 2 out]
        n94 = property class="DigNum (strict)"(reference=w244, "Value"=0) -> ()  [unwired: 1 in, 2 out]
        n95 = Bundle("Value"=w253, "Value"=w252) -> (w251:cluster{"Value":timestamp, "Value":timestamp})  [unwired: 1 in]
        n96 = Empty String/Path?(string/path=w248) -> (empty?=w249:bool)
        n97 = case shown="False" w249 {
          tunnel: w258 -> [w266 w270]
          tunnel: w256 -> [w265 w269]
          tunnel: w251 -> [w263 w268]
          tunnel: w248 -> [w264 _]
          tunnel: [w262 w267] -> w246
          frame False {
            n98 = call-poly <vilib>:"Query Data.vi"("Time Range"=w263, "Serial Number"=w264, "Sequence Name"=w265, "Database Configuration"=w266) -> ("Data"=w262:T5)  [unwired: 6 in, 1 out]
          }
          frame True {
            n99 = call-poly <vilib>:"Query Data.vi"("Time Range"=w268, "Sequence Name"=w269, "Database Configuration"=w270) -> ("Data"=w267:T5)  [unwired: 7 in, 1 out]
          }
        }
        n100 = Bundle By Name(cluster=w247, "Data"=w246) -> (w245:T4)
        n101 = call <vilib>:"Add State(s) to Queue__JKI_lib_State_Machine.vi"("State(s) in (\"\")"=w261) -> ("States Out"=w260:string)  [unwired: 14 in]
      }
      frame "Data Query: Show Data" {
        # "Your code here.\n(You can make a copy of, or modify, this frame)"
        n102 = Unbundle By Name(w277) -> ("Listbox"=w276:refnum<vi>, "Data"=w275:T5, "Page"=w273:refnum<vi>)
        n103 = property class="DigNum (strict)"(reference=w273) -> ("Value"=w272:i32)  [unwired: 1 in, 2 out]
        n104 = Reverse 1D Array(array=w275) -> (reversed array=w271:T5)
        n105 = call "Select Data Items.vi"("Page"=w272, "Data"=w271) -> ("subarray"=w274:string[][])  [unwired: 9 in]
        n106 = property class="MCListbox (strict)"(reference=w276, "ItemNames"=w274) -> ()  [unwired: 1 in, 2 out]
        n107 = call <vilib>:"Add State(s) to Queue__JKI_lib_State_Machine.vi"("State(s) in (\"\")"=w280) -> ("States Out"=w279:string)  [unwired: 14 in]
      }
      frame "Data Query: Detailed" {
        # "Template Separator\n(You can make a copy of, or modify, this frame)"
        n108 = Unbundle By Name(w299) -> ("Data"=w292:T5, "Page"=w298:refnum<vi>, "Listbox"=w295:refnum<vi>)
        n109 = property class="DigNum (strict)"(reference=w298) -> ("Value"=w297:i32)  [unwired: 1 in, 2 out]
        n110 = property class="MCListbox (strict)"(reference=w295) -> ("Value"=w294:i32)  [unwired: 1 in, 2 out]
        n111 = Multiply(x=w297, y=24) -> (x*y=w281:i32)
        n112 = vi-ref "Detailed Data.vi"() -> (w287:refnum<vi>)
        n113 = Add(x=w281, y=w294) -> (x+y=w290:i32)
        n114 = property class="VI"(reference=w287) -> ("Name"=w286:string)  [unwired: 1 in, 2 out]
        n115 = Index Array(array=w292, index=w290) -> (element=w293:T7)
        n116 = Less Than 0?(x=w290) -> (x < 0?=w289:bool)
        n117 = Empty Array?(array=w292) -> (empty?=w291:bool)
        n118 = Open VI Reference(type specifier VI Refnum (for type only)=refnum<vi> refnum, vi path=w286, options=128) -> (vi reference=w283:refnum<vi>)  [unwired: 3 in, 1 out]
        n119 = Or(x=w291, y=w289) -> (x .or. y?=w288:bool)
        n120 = case shown="True" w288 {
          tunnel: w293 -> [w304 _]
          tunnel: w283 -> [w305 w306]
          tunnel: [w303 w306] -> w282
          frame False {
            n121 = call-by-ref "Start Asynchronous Call"(reference=w305, "Data"=w304) -> (reference out=w303:refnum<vi>)  [unwired: 12 in, 1 out]
          }
          frame True {
          }
        }
        n122 = Close Reference(reference=w282) -> ()  [unwired: 1 in, 1 out]
        n123 = call <vilib>:"Add State(s) to Queue__JKI_lib_State_Machine.vi"("State(s) in (\"\")"=w302) -> ("States Out"=w301:string)  [unwired: 14 in]
      }
      frame "Data Query: Next Page" {
        # "Do not put any code in this frame.\n(It is a separator no-op. You can make a copy of this frame to create a new Data frame)"
        n124 = Unbundle By Name(w317) -> ("Data"=w314:T5, "Page"=w316:refnum<vi>)
        n125 = Array Size(array=w314) -> (size(s)=w313:i32)
        n126 = property class="DigNum (strict)"(reference=w316) -> (reference out=w309:refnum<vi>, "Value"=w315:i32)  [unwired: 1 in, 1 out]
        n127 = Quotient & Remainder(x=w313, y=24) -> (floor(x/y)=w311:i32)  [unwired: 1 out]
        n128 = Increment(x=w315) -> (x+1=w308:i32)
        n129 = Greater?(x=w308, y=w311) -> (0:w310:bool)
        n130 = case shown="False" w310 {
          tunnel: w309 -> [w323 _]
          tunnel: w308 -> [w322 _]
          tunnel: ["Data Query: Show Data" ("State(s) at Back (\"\")") _] -> w307
          frame False {
            n131 = property class="DigNum (strict)"(reference=w323, "Value"=w322) -> ()  [unwired: 1 in, 2 out]
          }
          frame True {
          }
        }
        n132 = call <vilib>:"Add State(s) to Queue__JKI_lib_State_Machine.vi"("State(s) in (\"\")"=w320, "State(s) at Back (\"\")"=w307) -> ("States Out"=w319:string)  [unwired: 13 in]
      }
      frame "Data Query: Previous Page" {
        # "Do not put any code in this frame.\n(It is a separator no-op. You can make a copy of this frame to create a new Data frame)"
        n133 = Unbundle By Name(w327) -> ("Page"=w330:refnum<vi>)
        n134 = property class="DigNum (strict)"(reference=w330) -> (reference out=w329:refnum<vi>, "Value"=w328:i32)  [unwired: 1 in, 1 out]
        n135 = Decrement(x=w328) -> (x-1=w325:i32)
        n136 = Less Than 0?(x=w325) -> (x < 0?=w324:bool)
        n137 = case shown="False" w324 {
          tunnel: w329 -> [w336 _]
          tunnel: ["Data Query: Show Data" ("State(s) at Back (\"\")") _] -> w326
          tunnel: w325 -> [w334 _]
          frame False {
            n138 = property class="DigNum (strict)"(reference=w336, "Value"=w334) -> ()  [unwired: 1 in, 2 out]
          }
          frame True {
          }
        }
        n139 = call <vilib>:"Add State(s) to Queue__JKI_lib_State_Machine.vi"("State(s) in (\"\")"=w333, "State(s) at Back (\"\")"=w326) -> ("States Out"=w332:string)  [unwired: 13 in]
      }
      frame "Data Query: Export" {
        # "Template Separator\n(You can make a copy of, or modify, this frame)"
        n140 = disable-structure shown="Disabled" {
          disable-tunnel: w337 -> [w349 _]
          frame Disabled {
            w348 = T8 2 items=["User Home"=0, "User Desktop"=1, "User Documents"=2, "User Application Data"=3, "User Preferences"=4, "User Temporary"=5, "Public Documents"=6, "Public Application Data"=7, "Public Preferences"=8, "Public Cache"=13, "System Core Libraries"=9, "System Installed Libraries"=10, "Application Files"=11, "Boot Volume Root"=12] ("system directory type")
            n141 = call <vilib>:"Get System Directory.vi"("system directory type"=w348) -> ("system directory"=w347:path)  [unwired: 10 in]
            n142 = Unbundle By Name(w349) -> ("Data"=w345:T5)
            n143 = call "File Dialog"("start path"=w347, "pattern (all files)"="*.xlsx") -> ("selected path"=w344:path, "cancelled"=w343:bool, "error out"=w342:errorcluster)  [unwired: 10 in, 1 out]
            n144 = Or(x=w343, y=w342) -> (x .or. y?=w341:bool)
            n145 = case shown="False" w341 {
              tunnel: w345 -> [w356 _]
              tunnel: w344 -> [w355 _]
              frame False {
                n146 = Two Button Dialog(message="是否需要添加详细数据工作表。", 1:"不需要" ("F button name (\"Cancel\")"), 2:"需要" ("T button name (\"OK\")")) -> (T button?=w352:bool)
                n147 = call-poly <vilib>:"Query Data.vi"("Adding Detailed Data"=w352, "Save to file"=TRUE, "report file path"=w355, "Data"=w356) -> ()  [unwired: 5 in, 3 out]
              }
              frame True {
              }
            }
          }
          frame Enabled {
          }
        }
        n148 = call <vilib>:"Add State(s) to Queue__JKI_lib_State_Machine.vi"("State(s) in (\"\")"=w340) -> ("States Out"=w339:string)  [unwired: 14 in]
      }
      frame "Data Query: Goto" {
        # "Template Separator\n(You can make a copy of, or modify, this frame)"
        n149 = Unbundle By Name(w363) -> ("Data"=w368:T5, "Page"=w362:refnum<vi>)
        n150 = Scan From String(format string="%d,%d", input string=w359) -> (output 1=w357:i32, output 2=w358:i32)  [unwired: 4 in, 3 out]
        n151 = Array Size(array=w368) -> (size(s)=w367:i32)
        n152 = Quotient & Remainder(x=w367, y=24) -> (floor(x/y)=w365:i32)  [unwired: 1 out]
        n153 = Greater?(x=w358, y=w365) -> (0:w364:bool)
        n154 = case shown="True" w364 {
          tunnel: w362 -> [w374 w376]
          tunnel: w358 -> [w373 _]
          tunnel: ["Data Query: Show Data" ("State(s) at Back (\"\")") _] -> w361
          tunnel: w357 -> [_ w375]
          frame False {
            n155 = property class="DigNum (strict)"(reference=w374, "Value"=w373) -> ()  [unwired: 1 in, 2 out]
          }
          frame True {
            n156 = property class="DigNum (strict)"(reference=w376, "Value"=w375) -> ()  [unwired: 1 in, 2 out]
          }
        }
        n157 = call <vilib>:"Add State(s) to Queue__JKI_lib_State_Machine.vi"("State(s) in (\"\")"=w371, "State(s) at Back (\"\")"=w361) -> ("States Out"=w370:string)  [unwired: 13 in]
      }
    }
  }
  "Error Out" <- w3
